vi "Generator.Synthesize Waveforms.vi"(0 "Generator.lvclass":refnum<class "Generator.lvclass">, 5 "sweep state":T1, 11 "error in (no error)":errorcluster, 12 "Reset Phase?":bool) -> (4 "Generator.lvclass":refnum<class "Generator.lvclass">, 6 "AO waveform":waveform(dbl)[](array[waveform]), 8 "X waveforms":waveform(dbl)[](array[waveform]), 10 "Y waveforms":waveform(dbl)[](array[waveform]), 15 "error out":errorcluster)   [LabVIEW 2019, in "Generator.lvclass"]
uses:
  Generator.lvclass
  Instrument.DAQ/Typedefs/Sweep.State--enum.ctl
  Instrument.DAQ/Instrument.DAQ.lvclass
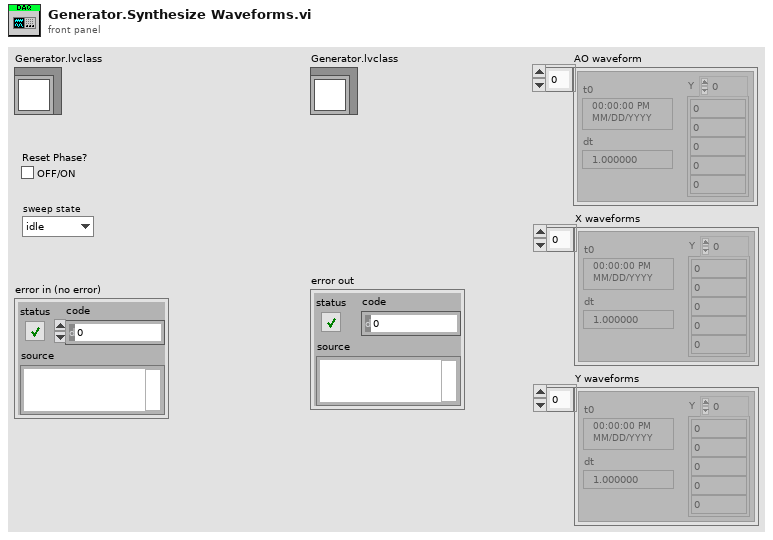
[diagram p1: front panel]
types:
  T1 = typedef "Instrument.Lockin.lvlib/Instrument.DAQ.lvclass/Sweep.State--enum.ctl" = enum16{"idle", "initialize", "wait", "sweep", "stop"}
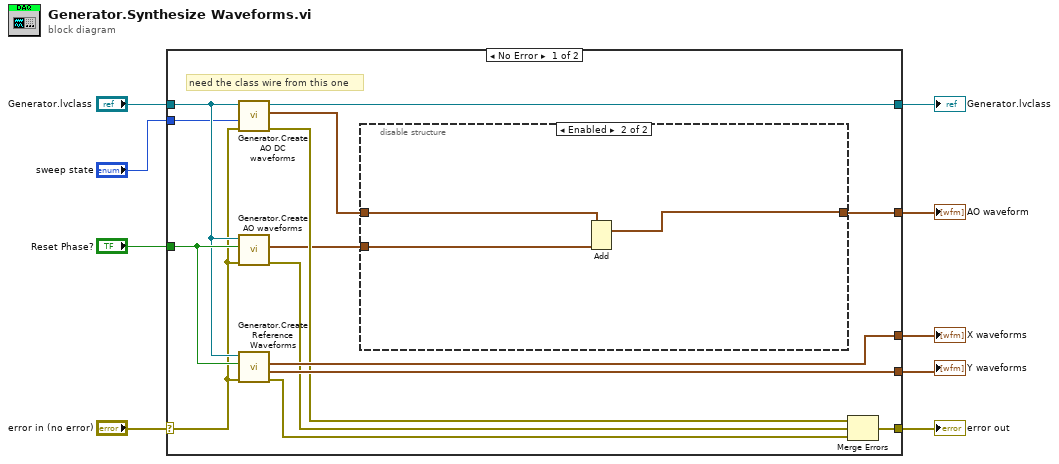
[diagram p0: block diagram]
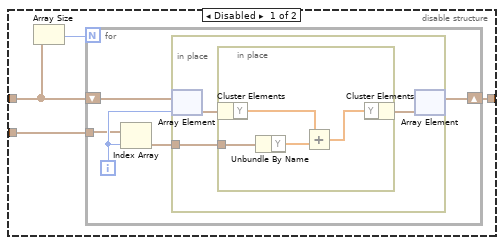
[diagram p2: hidden frame]
diagram:
  n1 = case shown="No Error" "error in (no error)" {
    selector: "error in (no error)" -> [w15 w44]
    tunnel: [w16 _] -> w2
    tunnel: "Reset Phase?" -> [w23 _]
    tunnel: [w10 _] -> w3
    tunnel: [w22 w44] -> w8
    tunnel: "Generator.lvclass" -> [w21 w43]
    tunnel: "sweep state" -> [w17 _]
    tunnel: [w19 w43] -> w4
    tunnel: [w18 _] -> w1
    frame No Error {
      # "need the class wire from this one"
      n2 = call "Generator.Create AO DC waveforms.vi"("error in (no error)"=w15, "sweep state"=w17, "Generator in"=w21) -> ("error out"=w13:errorcluster, "AO Array"=w11:waveform(dbl)[], "Generator out"=w19:refnum<class "Generator.lvclass">)  [unwired: 6 in]
      n3 = call "Generator.Create AO waveforms.vi"("error in (no error)"=w15, "reset phase"=w23, "Generator in"=w21) -> ("error out"=w14:errorcluster, "AO Array"=w12:waveform(dbl)[])  [unwired: 6 in, 1 out]
      n4 = call "Generator.Create Reference Waveforms.vi"("error in (no error)"=w15, "reset phase"=w23, "Generator in"=w21) -> ("error out"=w20:errorcluster, "Y"=w18:waveform(dbl)[], "X"=w16:waveform(dbl)[])  [unwired: 4 in, 2 out]
      n5 = disable-structure shown="Enabled" {
        disable-tunnel: w12 -> [w27 w41]
        disable-tunnel: w11 -> [w24 w42]
        disable-tunnel: [w25 w40] -> w10
        frame Disabled {
          n6 = Array Size(array=w24) -> (size(s)=w26:i32)
          n7 = for {
            N: w26 -> [_]
            shift-right: [w30] -> w25
            shift-left: w24 -> [w28]
            tunnel: w27 -> [w29]
            i -> [w32]
            n8 = Index Array(array=w29, index=w32) -> (element=w31:waveform(dbl))
            n9 = in-place {
              in-place-border: w31 -> [w34]
              n10 = in-place-array #1(w28, w32) -> (w35:waveform(dbl))
              n11 = in-place {
                in-place-border: w34 -> [w38]
                n12 = in-place-cluster #2(w35) -> ("Y"=w37:dbl[])
                n13 = Unbundle By Name(w38) -> ("Y"=w36:dbl[])
                n14 = Add(x=w37, y=w36) -> (x+y=w39:dbl[])
                n15 = in-place-cluster #2("Y"=w39) -> (w33:waveform(dbl))
              }
              n16 = in-place-array #1(w33) -> (w30:waveform(dbl)[])  [unwired: 1 out]
            }
          }
        }
        frame Enabled {
          n17 = Add(1:w41, 2:w42) -> (0:w40:waveform(dbl)[])  [unwired: 1 in, 1 out]
        }
      }
      n18 = Merge Errors(w13, w14, w20) -> (w22:errorcluster)
    }
    frame Error {
    }
  }
  "error out" <- w8
  "Generator.lvclass" <- w4
  "AO waveform" <- w3
  "X waveforms" <- w2
  "Y waveforms" <- w1
